vi "Write Cycle - Multiple DUTs - Common Data.vi"(0 "Cycle Instructions":T1[](array[typedef]) {"Post CMD Delay (s)" format="%#_4ps"; "DAC Vout (V)" format="%.3f V"; "Dev Ch Idx (0-5)" max=5 step=1 format="Ch %d"}, 11 "error in":errorcluster, 12 "FPGA":T2, 13 "Dev Mask (All)":bool[](array[boolean])=[TRUE, TRUE, TRUE, TRUE, TRUE, TRUE], 14 "Log (T)":bool=TRUE) -> (15 "error out":errorcluster)   [LabVIEW 2017, in "Host SRL.lvlib"]
uses:
  Host SRL.lvlib
  Type Defs/WSVCAP SHL FPGA Enum.ctl
  Type Defs/Cycle Instruction Cluster.ctl
panel:
  out "Socket Mask":u32=1 format="%02x"
  out "SRL Data Out [U8]":u8[][](array[numeric]) format="%02x"
  # "Dev 01"
  # "Dev 02"
  # "Dev 03"
  # "Dev 04"
  # "Dev 05"
  # "Dev 06"
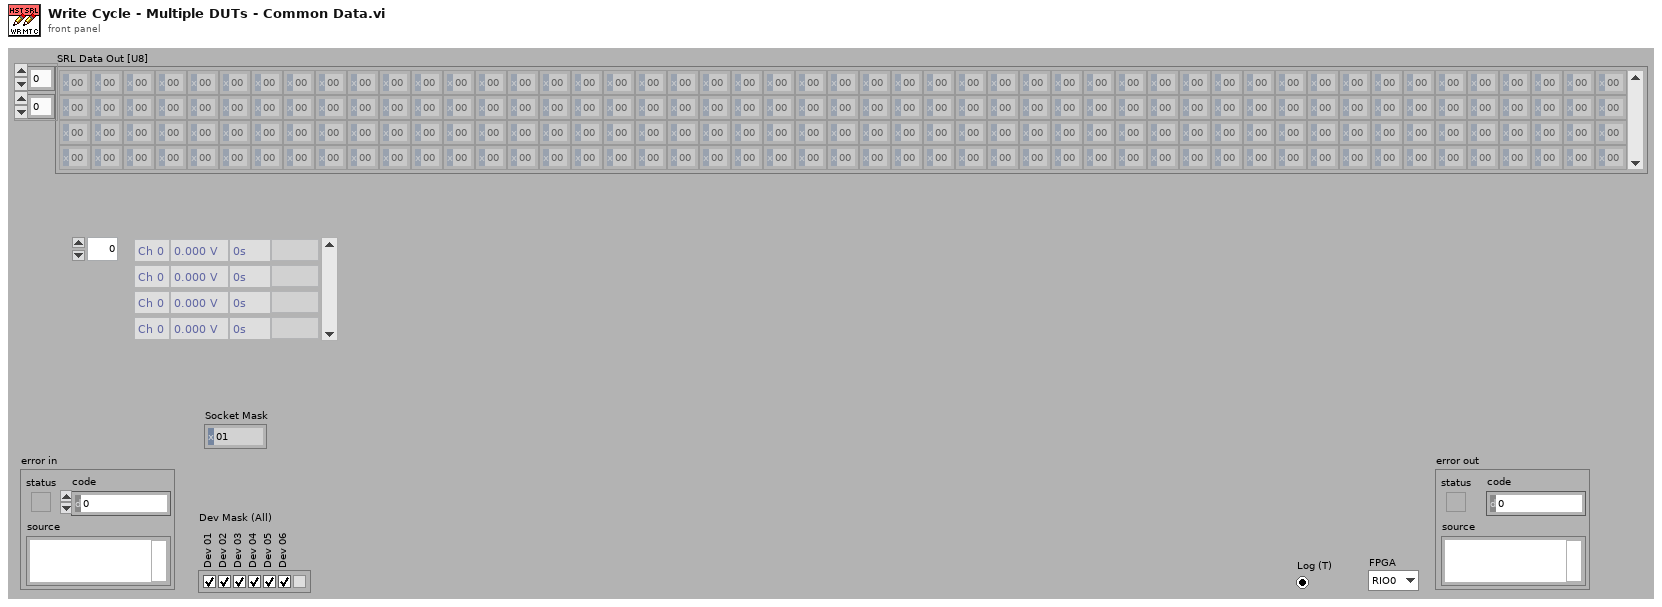
[diagram p1: front panel]
types:
  T1 = typedef "Host SRL.lvlib/Cycle Instruction Cluster.ctl" = cluster{"Dev Ch Idx (0-5)":u32, "DAC Vout (V)":dbl, "Post CMD Delay (s)":dbl, "Raw CMD":string}
  T2 = typedef "WSVCAP SHL FPGA Enum.ctl" = enum16{"RIO0", "RIO1"}
  T3 = typedef "WSVCAP SHL Core System Cluster.ctl" = cluster{"Settings":T4, "FPGA Resource":tag, "Online":bool, "I2C Wait Ticks":u32, "SRL Wait Ticks":u32, "FPGA VI Reference (FPGA Mode)":T5, "FPGA VI Reference (Sim Mode)":refnum<vi>}
  T4 = typedef "WSVCAP SHL I2C Settings Cluster.ctl" = cluster{"I2C Slave Address":u8, "I2C Clock Rate (Hz)":dbl, "SRL Clock Rate (Hz)":dbl, "Simulate FPGA":bool, "C1 Cap DAC Default":u8, "C2 Cap DAC Default":u8, "C3 Cap DAC Default":u8, "C4 Cap DAC Default":u8, "DAC Out Vref (V)":dbl}
  T5 = typedef "WSVCAP SHL FPGA Ref.ctl" = refnum<k20>
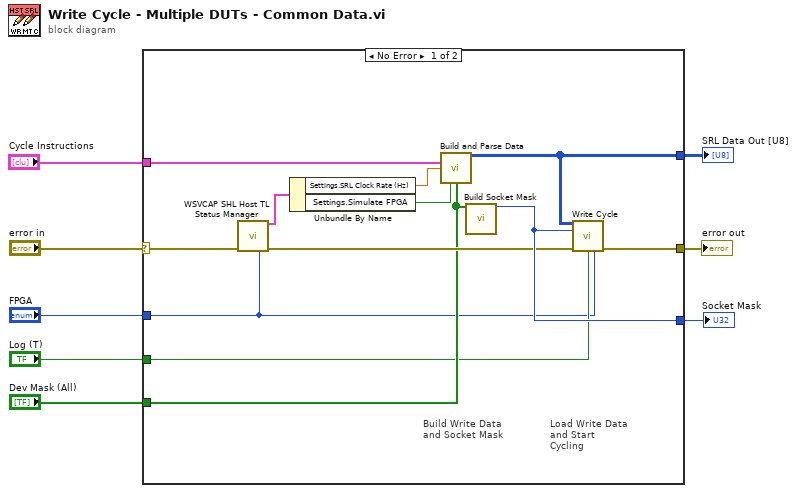
[diagram p0: block diagram]
diagram:
  n1 = case shown="No Error" "error in" {
    selector: "error in" -> [w10 _]
    tunnel: [w20 _] -> w8
    tunnel: [w19 _] -> w6
    tunnel: [w18 _] -> w5
    tunnel: "Dev Mask (All)" -> [w13 _]
    tunnel: "Log (T)" -> [w12 _]
    tunnel: "FPGA" -> [w11 _]
    tunnel: "Cycle Instructions" -> [w9 _]
    frame No Error {
      # "Load Write Data and Start Cycling"
      # "Build Write Data and Socket Mask"
      n2 = call "WSVCAP SHL Host TL Status Manager.vi"("error in"=w10, "FPGA"=w11) -> ("System Out"=w17:T3, "error out"=w16:errorcluster)  [unwired: 12 in]
      n3 = Unbundle By Name(w17) -> ("Settings.SRL Clock Rate (Hz)"=w14:dbl, "Settings.Simulate FPGA"=w15:bool)
      n4 = call "Build and Parse Data.vi"("Cycle Instructions"=w9, "Clock Rate (Hz) (Cycle Only)"=w14, "Simulate FPGA (Cycle Only)"=w15, "Dev Mask (All)"=w13) -> ("SRL Data Out [U8]"=w19:u8[][])  [unwired: 10 in, 1 out]
      n5 = call "Build Socket Mask.vi"("Dev Mask (All)"=w13) -> ("Socket Mask [U32]"=w18:u32)  [unwired: 14 in]
      n6 = call "Write Cycle.vi"("SRL Data Out"=w19, "Socket Mask"=w18, "error in"=w16, "Log (T)"=w12, "FPGA"=w11) -> ("error out"=w20:errorcluster)  [unwired: 10 in]
    }
    frame Error {
    }
  }
  "error out" <- w8
  "SRL Data Out [U8]" <- w6
  "Socket Mask" <- w5
